vi "Gyro PID Fwd C4 Assisted - Right Edge.vi"(5 "Target reflection":sgl=32.0, 6 "Target angle":sgl, 7 "Threshold to Color":i32=1200, 8 "Threshold to slow":i32=1000, 9 "Min. speed":i32=20, 10 "Max. speed":i32=40, 11 "EV3 in":T1) -> (3 "EV3 out":T1)   [LabVIEW 2016]
uses:
  <vilib>/NXT/Subs/LVHSConnector.ctl
  <vilib>/NXT/LegoClasses/BrickReference/BrickReference.lvclass
  <vilib>/NXT/Block Support/NXT_OutputPort.ctl
  <vilib>/NXT/Block Support/NXT_InputPort.ctl
  <vilib>/NXT/NXTIO Xnodes/NXTIONodeSubVIs/LEGOResetMotors.vi
  <vilib>/NXT/Dual Mode Library/Motors/Rotation.vi
  <vilib>/NXT/Dual Mode Library/Sensors/EV3_Color_Reflect.vi
  <vilib>/NXT/NXTIO Xnodes/NXTIONodeSubVIs/NXTMotorSteeringOn.vi
  <vilib>/NXT/NXTIO Xnodes/NXTIONodeSubVIs/NXTStopMotors.vi
  <vilib>/NXT/Dual Mode Library/Waits/Wait_Num.vi
  <vilib>/NXT/NXTIO Xnodes/NXTIOXNode/NXTIO.xnode
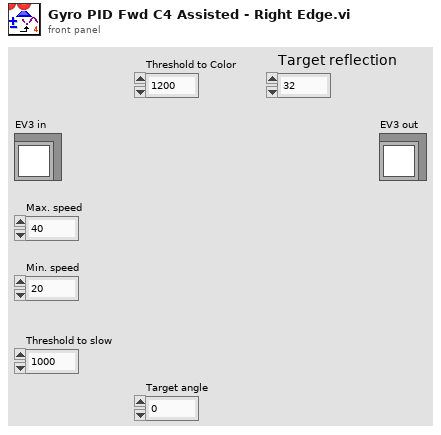
[diagram p1: front panel]
types:
  T1 = typedef "LVHSConnector.ctl" = refnum<class "BrickReference.lvclass">
  T2 = typedef "NXT_OutputPort.ctl" = u8
  T3 = typedef "NXT_InputPort.ctl" = u32
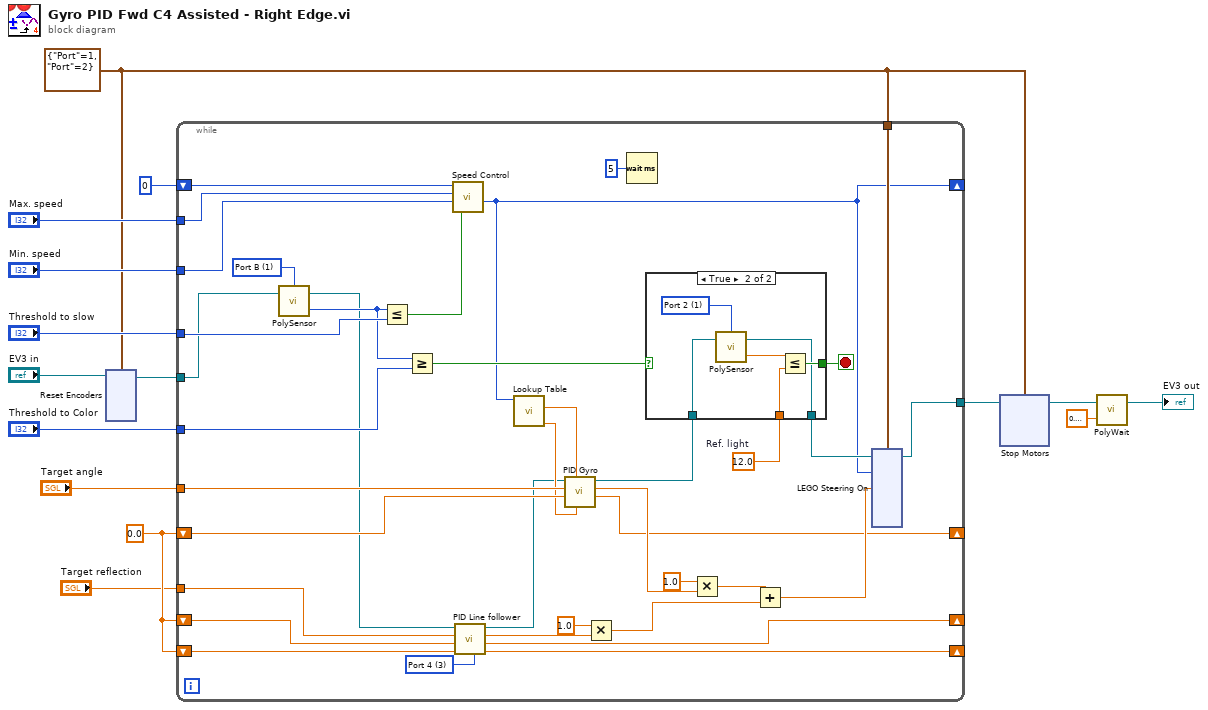
[diagram p0: block diagram]
diagram:
  w6 = cluster{"Port":T2, "Port":T2} {"Port"=1, "Port"=2} ("Motor")
  w2 = sgl 0.0
  n1 = xnode "Reset Encoders"("Motors"=w6, "NXT/EV3"="EV3 in") -> ("NXT/EV3"=w12:T1)
  n2 = while {
    tunnel: w12 -> [w44]
    shift-right: [w19] -> _
    shift-left: w2 -> [w41]
    tunnel: "Target angle" -> [w53]
    tunnel: [w50] -> w8
    tunnel: w6 -> [w52]
    shift-right: [w32] -> _
    shift-left: 0 -> [w48]
    tunnel: "Min. speed" -> [w45]
    tunnel: "Max. speed" -> [w47]
    tunnel: "Threshold to slow" -> [w46]
    tunnel: "Threshold to Color" -> [w40]
    shift-right: [w25] -> _
    shift-left: w2 -> [w29]
    shift-right: [w26] -> _
    shift-left: w2 -> [w27]
    tunnel: "Target reflection" -> [w23]
    stop <- w39 stop-if-true
    w16 = T3 3 items=["Port 1", "Port 2", "Port 3", "Port 4"] ("Port (Port 1)")
    w35 = sgl 12.0  # Ref. light
    w51 = T2 1 items=["Port A", "Port B", "Port C", "Port D"] ("Port (Port A)")
    n3 = call-poly <vilib>:"PolySensor.vi"("NXT/EV3"=w44, "Port (Port A)"=w51) -> ("Angle of Rotation"=w42:i32, "NXT/EV3"=w22:T1)  [unwired: 1 in]
    n4 = Less Or Equal?(x=w42, y=w46) -> (x <= y?=w43:bool)
    n5 = Greater Or Equal?(x=w42, y=w40) -> (x >= y?=w38:bool)
    n6 = call "Speed Control.vi"("Speed Up or Down?"=w43, "Min. speed"=w45, "Max. speed"=w47, "Ini. speed"=w48) -> ("Speed out"=w32:i32)  [unwired: 7 in]
    n7 = call "PID Line follower.vi"("Port (Port 1)"=w16, "Old Error"=w29, "Previous integral"=w27, "Target reflection"=w23, "EV3 in"=w22) -> ("New Error"=w25:sgl, "New integral"=w26:sgl, "Total error"=w24:sgl, "EV3 out"=w28:T1)  [unwired: 3 in]
    n8 = call "Lookup Table.vi"("Speed"=w32) -> ("I"=w30:dbl, "P"=w31:dbl)  [unwired: 9 in]
    n9 = call "PID Gyro.vi"("K_i"=w30, "K_p"=w31, "Previous integral"=w41, "Target angle"=w53, "EV3 in"=w28) -> ("New integral"=w19:sgl, "Total error"=w34:sgl, "EV3 out"=w37:T1)  [unwired: 4 in]
    n10 = Multiply(x=sgl 1.0, y=w24) -> (x*y=w21:sgl)
    n11 = Wait (ms)(milliseconds to wait=u32 5) -> ()  [unwired: 1 out]
    n12 = case shown="True" w38 {
      tunnel: [_ w58] -> w39
      tunnel: w37 -> [w54 w57]
      tunnel: [w54 w56] -> w36
      tunnel: w35 -> [_ w55]
      frame False {
      }
      frame True {
        w60 = T3 1 items=["Port 1", "Port 2", "Port 3", "Port 4"] ("Port (Port 1)")
        n13 = call-poly <vilib>:"PolySensor.vi"("NXT/EV3"=w57, "Port (Port 1)"=w60) -> ("Scaled Value"=w59:sgl, "NXT/EV3"=w56:T1)  [unwired: 1 in]
        n14 = Less Or Equal?(x=w59, y=w55) -> (x <= y?=w58:bool)
      }
    }
    n15 = Multiply(x=sgl 1.0, y=w34) -> (x*y=w18:sgl)
    n16 = Add(x=w18, y=w21) -> (x+y=w33:sgl)
    n17 = xnode "LEGO Steering On"("Steering 1"=w33, "Power 1"=w32, "Motors"=w52, "NXT/EV3"=w36) -> ("NXT/EV3"=w50:T1)
  }
  n18 = xnode "Stop Motors"("Motors"=w6, "NXT/EV3"=w8) -> ("NXT/EV3"=w7:T1)
  n19 = call-poly <vilib>:"PolyWait.vi"("Time (1 sec)"=sgl 0.2, "NXT/EV3"=w7) -> ("NXT/EV3"=→"EV3 out":T1)  [unwired: 2 in]
